vi "PH_PPMA_PowerUnit.src Voltage.vi"(0 "i ref in":refnum<vi>, 2 "Voltage [V]":dbl, 5 "error in (no error)":errorcluster) -> (14 "i ref out":refnum<vi>, 19 "error out":errorcluster)   [LabVIEW 2014, in "PH_PPMA_PowerUnit.lvlib"]
doc: "This is the action VI of the Set Voltage event case. It checks whether the SM State is \"Switch PU on\" or \"Wait for Shot Cmd\" and HV off = false and Ignitron Device State = on. If this is true, it coeres the incoming voltage to the allowed range and writes it to the attributes. The voltage is written to the attributes of the SM and a state change request is send to SM for \"Set Settings\"."
uses:
  PH_PPMA_PowerUnit.lvlib
  PH_StatusHandler/PH_StatusHandler.Status.ctl
  PH_PowerUnit_BaseClass/PH_PowerUnit_BaseClass.SM States.ctl
  CSCore/BaseSM/BaseSM.lvlib
  PH_Common/PH_Common.lvlib
  PH_PowerUnit_BaseClass/PH_PowerUnit_BaseClass.lvlib
  PH_StatusHandler/PH_StatusHandler.lvlib
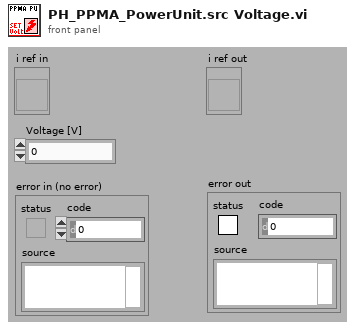
[diagram p1: front panel]
types:
  T1 = typedef "PH_PowerUnit_BaseClass.lvlib/PH_PowerUnit_BaseClass.i attribute.ctl" = cluster{"Constructor finished":bool, "PU":cluster{"In use":bool, "Service ID in use":i32, "GUI Ref":refnum<vi>}, "Enabling":cluster{"State":T2, "GUI Ref":refnum<vi>}, "Timing":cluster{"Last Shot":dbl, "Time between Shots [Sec]":dbl, "Waiting Time over?":bool, "Service ID Waiting Time":i32, "GUI Ref":refnum<vi>, "Instance":cluster{"Status":T3, "linked?":bool, "GUI Ref":refnum<vi>}}, "Sequencer":cluster{"SM State":string, "GUI Ref":refnum<vi>, "linked":bool}, "Subscribed Trendmssgs":cluster{"Tagname":string, "Status":T3, "linked?":bool, "Shot Condition":T3, "GUI Ref":refnum<vi>}[], "PP PU":T4, "Default Voltage (V)":dbl, "GUI Refs":T5, "PSDB data":cluster{"Shot Voltage [V]":dbl, "State TO SM":T6, "Write 2 early":bool}, "State TO SM":T6}
  T2 = typedef "PH_SystemInformation.lvlib/PH_SystemInformationEnabling State.ctl" = i32
  T3 = typedef "PH_StatusHandler.lvlib/PH_StatusHandler.Status.ctl" = i16
  T4 = typedef "PH_PP_Common.lvlib/PH_PP_Common.PUs.ctl" = enum16{"no Info", "PA-19mm-1", "PA-19mm-2", "PA-45mm-PILC", "PA-45mm-MAIN", "MA-PU-1", "MA-PU-2", "MA-PU-3", "MA-PU-4", "MA-PU-5", "MA-PU-6", "MA-FR", "MA-PILC", "PA-45mm-DP"}
  T5 = typedef "PH_PowerUnit_BaseClass.lvlib/PH_PowerUnit_BaseClass.GUI Refs.ctl" = cluster{"Delete Inst":refnum<vi>, "State TO SM":refnum<vi>, "State SM":refnum<vi>, "Fire":refnum<vi>}
  T6 = typedef "PH_PowerUnit_BaseClass.lvlib/PH_PowerUnit_BaseClass.SM States.ctl" = enum16{".", "Stand by", "Switch PU on", "Configure", "Set Default Voltage", "Set STANDBY", "Set READY", "Wait for Shot Cmd", "Open Dump Rods", "Open Ross Relais", "Close Ross Relais", "Switch PSU on", "Switch PSU off", "Charge", "Switch GD Channel on", "Close Dump Rods", "Rods-TO", "RR-TO", "PSU-TO", "Trigger-TO"}
  T7 = typedef "PH_PPMA_PowerUnit.lvlib/PH_PPMA_PowerUnit.i attribute.ctl" = cluster{"GUI Refs":cluster{"Rods":refnum<vi>, "Ignitron":refnum<vi>, "Rossrelais":refnum<vi>, "Set Voltage":refnum<vi>, "PSU":refnum<vi>, "EOC":refnum<vi>, "Trigger":refnum<vi>}, "Rods":T8, "PSU":T9, "Ross Relais":T10, "Ignitron":T11, "Trigger":cluster{"State Device":T3, "linked?":bool}, "Timing Settings":cluster{"Prdc Fast?":bool, "Default Value Periodic Interval":i32, "Mercury on since":dbl, "Warm up Time Mercury [s]":dbl}, "Set Voltage [V]":dbl}
  T8 = typedef "PH_PPMA_PowerUnit.lvlib/PH_PPMA_PowerUnit.Rods Attributes.ctl" = cluster{"Instancename":string, "Device Status":T3, "linked?":bool}
  T9 = typedef "PH_PP_Common.lvlib/PH_PP_Common.PSU Attributes.ctl" = cluster{"lower limit [V]":dbl, "upper limit [V]":dbl, "Voltage set":bool, "State Device":T3, "linked?":bool}
  T10 = typedef "PH_PP_Common.lvlib/PH_PP_Common.Ross Relais Attributes.ctl" = cluster{"State Device":T3, "linked?":bool}
  T11 = typedef "PH_PP_Common.lvlib/PH_PP_Common.Ignitron Attributes.ctl" = cluster{"State Device":T3, "linked?":bool}
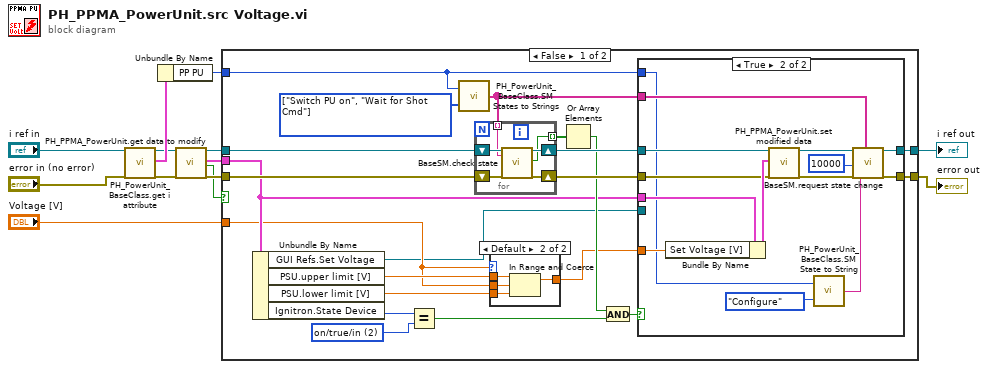
[diagram p0: block diagram]
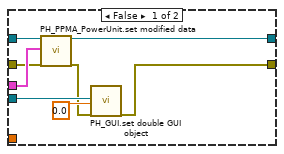
[diagram p3: hidden frame]
diagram:
  n1 = call "PH_PowerUnit_BaseClass.get i attribute.vi"("i ref in"="i ref in", "error in (no error)"="error in (no error)") -> ("i ref out"=w2:refnum<vi>, "i attribute"=w6:T1, "error out"=w4:errorcluster)  [unwired: 15 in]
  n2 = Unbundle By Name(w6) -> ("PP PU"=w1:T4)
  n3 = call "PH_PPMA_PowerUnit.get data to modify.vi"("i ref in"=w2, "error in (no error)"=w4) -> ("i ref out"=w11:refnum<vi>, "i attribute"=w13:T7, "timed out"=w8:bool, "error out"=w12:errorcluster)  [unwired: 14 in]
  n4 = case shown="False" w8 {
    tunnel: w13 -> [w24 _]
    tunnel: w12 -> [w32 w68]
    tunnel: w11 -> [w19 w69]
    tunnel: [w18 w69] -> w10
    tunnel: [w17 w68] -> w9
    tunnel: "Voltage [V]" -> [w23 _]
    tunnel: w1 -> [w14 _]
    frame False {
      w16 = T6[] [enum."Switch PU on", enum."Wait for Shot Cmd"] items=[".", "Stand by", "Switch PU on", "Configure", "Set Default Voltage", "Set STANDBY", "Set READY", "Wait for Shot Cmd", "Open Dump Rods", "Open Ross Relais", "Close Ross Relais", "Switch PSU on", "Switch PSU off", "Charge", "Switch GD Channel on", "Close Dump Rods", "Rods-TO", "RR-TO", "PSU-TO", "Trigger-TO"] ("SM States")
      w29 = T3 2 items=["no info", "off/false/out", "on/true/in", "Failure", "Alarm", "Status 1", "Status 2", "Status 3"] ("Ignitron.State Device")
      n5 = Unbundle By Name(w24) -> ("GUI Refs.Set Voltage"=w21:refnum<vi>, "PSU.upper limit [V]"=w25:dbl, "PSU.lower limit [V]"=w26:dbl, "Ignitron.State Device"=w30:T3)
      n6 = Equal?(x=w30, y=w29) -> (x = y?=w28:bool)
      n7 = call "PH_PowerUnit_BaseClass.SM States to Strings.vi"("SM States"=w16, "PU"=w14) -> ("SM State Strings"=w15:string[])
      n8 = for {
        shift-right: [w44] -> w31
        shift-left: w32 -> [w45]
        shift-right: [w43] -> w33
        shift-left: w19 -> [w42]
        tunnel: w15 -> [w41] mode=indexing
        tunnel: [w40] -> w34 mode=indexing
        n9 = call "BaseSM.check state.vi"("i ref in"=w42, "requestedState"=w41, "error in (no error)"=w45) -> ("i ref out"=w43:refnum<vi>, "OK"=w40:bool, "error out"=w44:errorcluster)  [unwired: 11 in, 3 out]
      }
      n10 = case shown="Default" w23 {
        tunnel: w26 -> [_ w39]
        tunnel: w25 -> [_ w38]
        tunnel: w23 -> [w35 w37]
        tunnel: [w35 w36] -> w22
        frame 0 {
        }
        frame Default {
          n11 = In Range and Coerce(upper limit=w38, x=w37, lower limit=w39) -> (coerced(x)=w36:dbl)  [unwired: 1 out]
        }
      }
      n12 = Or Array Elements(Boolean array=w34) -> (logical OR=w27:bool)
      n13 = And(x=w27, y=w28) -> (x .and. y?=w20:bool)
      n14 = case shown="True" w20 {
        tunnel: [w46 w67] -> w17
        tunnel: w33 -> [w52 w60]
        tunnel: w31 -> [w50 w59]
        tunnel: w15 -> [_ w66]
        tunnel: w24 -> [w53 w65]
        tunnel: w22 -> [_ w64]
        tunnel: w21 -> [w49 _]
        tunnel: [w51 w57] -> w18
        tunnel: w14 -> [_ w54]
        frame False {
          n15 = call "PH_PPMA_PowerUnit.set modified data.vi"("i ref in"=w52, "i attribute"=w53, "error in (no error)"=w50) -> ("i ref out"=w51:refnum<vi>, "error out"=w47:errorcluster)  [unwired: 15 in]
          n16 = call "PH_GUI.set double GUI object.vi"("GUI object Ref"=w49, "value"=0.0 ("Set Voltage [V]"), "error in (no error)"=w47) -> ("error out"=w46:errorcluster)  [unwired: 16 in]
        }
        frame True {
          n17 = Bundle By Name(cluster=w65, "Set Voltage [V]"=w64) -> (w62:T7)
          n18 = call "PH_PPMA_PowerUnit.set modified data.vi"("i ref in"=w60, "i attribute"=w62, "error in (no error)"=w59) -> ("i ref out"=w61:refnum<vi>, "error out"=w58:errorcluster)  [unwired: 15 in]
          n19 = call "PH_PowerUnit_BaseClass.SM State to String.vi"("SM State"=PH_PowerUnit_BaseClass.SM_States."Configure", "PU"=w54) -> ("SM State String"=w55:string)
          n20 = call "BaseSM.request state change.vi"("i ref in"=w61, "ms timeout (10000)"=10000 ("ms timeout (-1)"), "error in (no error)"=w58, "requested state"=w55, "allowed current states"=w66) -> ("i ref out"=w57:refnum<vi>, "error out"=w67:errorcluster)  [unwired: 11 in, 2 out]
        }
      }
    }
    frame True {
    }
  }
  "i ref out" <- w10
  "error out" <- w9
